vi "BenchConfig_GetFilePath.vi"(8 "error in (no error)":errorcluster) -> (0 "error out":errorcluster, 3 "BenchConfigFilePath":path)   [LabVIEW 2013]
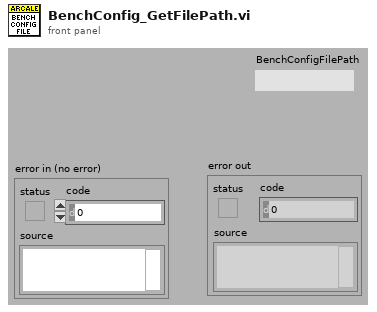
[diagram p1: front panel]
types:
  T1 = typedef "ApplicationPaths.ctl" = cluster{"Data Path":path, "Log Path":path, "Tmp Path":path}
  T2 = typedef "ApplicationInfos.ctl" = cluster{"ApplicationName":string, "ApplicationVersion":string, "Logo 600X200 path":path, "Logo 400X400 path":path, "Client":string}
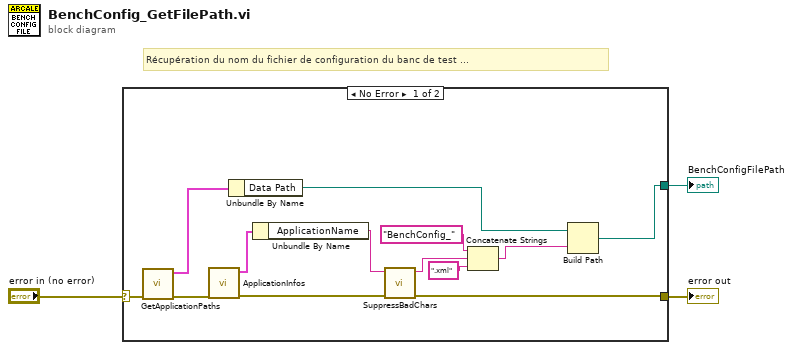
[diagram p0: block diagram]
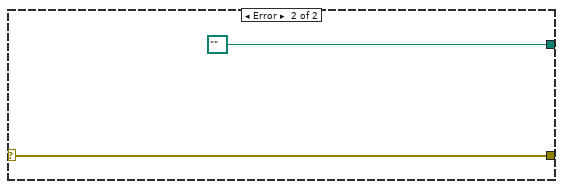
[diagram p2: hidden frame]
diagram:
  # "Récupération du nom du fichier de configuration du banc de test ..."
  n1 = case shown="No Error" "error in (no error)" {
    selector: "error in (no error)" -> [w15 w18]
    tunnel: [w4 w18] -> w2
    tunnel: [w9 path "" ("BenchConfigFilePath")] -> w1
    frame No Error {
      n2 = call "GetApplicationPaths.vi"("error in (no error)"=w15) -> ("error out"=w14:errorcluster, "ApplicationPath"=w13:T1)  [unwired: 9 in]
      n3 = call "ApplicationInfos.vi"("error in (no error)"=w14) -> ("error out"=w11:errorcluster, "ApplicationInfo"=w16:T2)  [unwired: 9 in]
      n4 = Unbundle By Name(w13) -> ("Data Path"=w10:path)
      n5 = Unbundle By Name(w16) -> ("ApplicationName"=w12:string)
      n6 = call "SuppressBadChars.vi"("error in (no error)"=w11, "StringIn"=w12) -> ("error out"=w4:errorcluster, "StringOut"=w8:string)  [unwired: 8 in]
      n7 = Concatenate Strings("BenchConfig_" ("string"), w8, ".xml" ("string")) -> (w5:string)
      n8 = Build Path(base path=w10, name or relative path=w5) -> (appended path=w9:path)
    }
    frame Error {
    }
  }
  "error out" <- w2
  "BenchConfigFilePath" <- w1
